vi "Create Bar Graph.vi"(9 "colors":u32[](array[colorbox]), 10 "names":string[](array[string]), 11 "values":dbl[](array[numeric])) -> (2 "Bar Graph":picture caption="Percentage of Test Gaps By Folder")   [LabVIEW 2009, in "GraphicalTestRunner.lvlib"]
uses:
  Graphical Test Runner/Graphical Test Runner Support/GraphicalTestRunner.lvlib
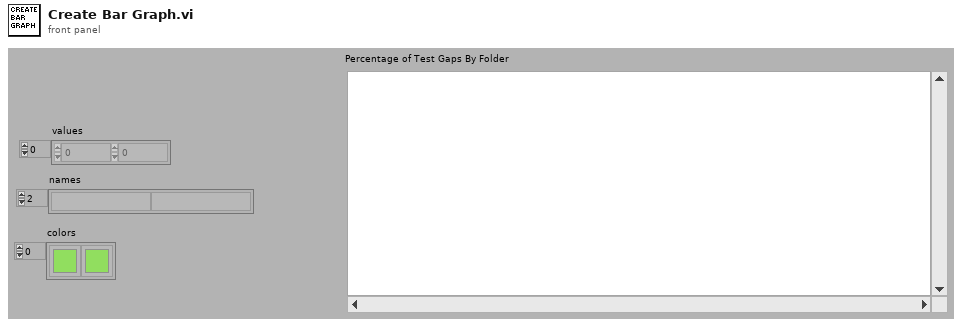
[diagram p1: front panel]
types:
  T1 = cluster{"horizontal":enum16{"left", "center", "right"}, "vertical":enum16{"top", "center", "bottom"}}
  T2 = cluster{"left":i16, "top":i16, "right":i16, "bottom":i16}
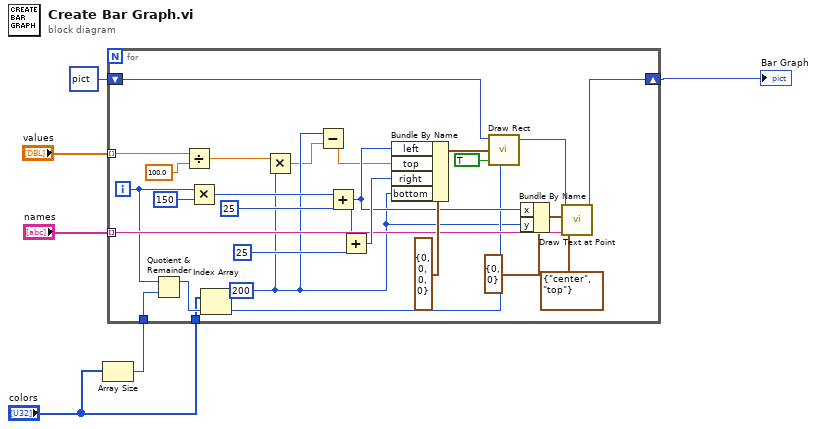
[diagram p0: block diagram]
diagram:
  n1 = Array Size(array="colors") -> (size(s)=w4:i32)
  n2 = for {
    tunnel: "values" -> [w19] mode=indexing
    tunnel: "names" -> [w25] mode=indexing
    tunnel: w4 -> [w14]
    tunnel: "colors" -> [w12]
    shift-right: [w23] -> w2
    shift-left: picture data[5B] ("new picture") -> [w10]
    i -> [w15]
    w9 = i16 200 ("bottom")
    n3 = Quotient & Remainder(x=w15, y=w14) -> (x-y*floor(x/y)=w13:i32)  [unwired: 1 out]
    n4 = Divide(x=w19, y=100.0 ("x")) -> (x/y=w18:dbl)
    n5 = Multiply(x=w15, y=150) -> (x*y=w31:i32)
    n6 = Index Array(array=w12, index=w13) -> (element=w11:u32)
    n7 = Multiply(x=w18, y=w9) -> (x*y=w8:dbl)
    n8 = Subtract(x=w9, y=w8) -> (x-y=w7:dbl)
    n9 = Add(x=w31, y=25) -> (x+y=w20:i32)
    n10 = Add(x=w20, y=25) -> (x+y=w28:i32)
    n11 = Bundle By Name(cluster=T2 {"left"=0, "top"=0, "right"=0, "bottom"=0} ("rect"), "left"=w20, "top"=w7, "right"=w28, "bottom"=w9) -> (w27:T2)
    n12 = call <vilib>:"Draw Rect.vi"("picture"=w10, "rect"=w27, "fill?(F)"=TRUE, "color(black)"=w11) -> ("new picture"=w24:picture)  [unwired: 5 in]
    n13 = Bundle By Name(cluster=cluster{"x":i16, "y":i16} {"x"=0, "y"=0} ("origin"), "x"=w20, "y"=w9) -> (w21:cluster{"x":i16, "y":i16})
    n14 = call <vilib>:"Draw Text at Point.vi"("text"=w25, "alignment(left, top)"=T1 {"horizontal"=enum."center", "vertical"=enum."top"}, "origin"=w21, "picture"=w24) -> ("new picture"=w23:picture)  [unwired: 6 in, 1 out]
  }
  "Bar Graph" <- w2
